vi "TPB Facade.vi"(0 "Data In":T5, 2 "Display State In":T2={"Window Handle"=refnum, "Maximum"=100, "State Change Action"=enum."Method - Initialize", "Running"=FALSE, "Visable Items"={"Label"=TRUE, "Caption"=FALSE}, "Value"=100, "Show Progress Bar"=FALSE}, 3 "Container State":T4) -> (6 "Data Out":T5, 7 "Display State Out":T2={"Window Handle"=refnum, "Maximum"=100, "State Change Action"=enum."Method - Initialize", "Running"=FALSE, "Visable Items"={"Label"=TRUE, "Caption"=FALSE}, "Value"=100, "Show Progress Bar"=FALSE}, 8 "Action":T1)   [LabVIEW 2011, in "Taskbar Progress Bar.xctl"]
uses:
  Taskbar Progress Bar.xctl
  TPB Data.ctl
  <vilib>/_xctls/Container State.ctl
  TPB State.ctl
  TypeDefs/Dispaly State Change Methods.ctl
  <vilib>/_xctls/Action.ctl
  <vilib>/TaskbarProgressAPI/_TypeDefs/Progress State.ctl
  <vilib>/_xctls/XControlSupport.lvlib
  <vilib>/TaskbarProgressAPI/TaskbarProgressAPI.lvlib
panel:
  out "Glyph":u16(ring)
  out "Progress Bar":u64(slide) scale=0.0..100.0
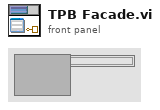
[diagram p1: front panel]
types:
  T1 = typedef "XControlSupport.lvlib/Action.ctl" = cluster{"Data Changed?":bool, "State Changed?":bool, "Action Name":string}
  T2 = typedef "Taskbar Progress Bar.xctl/TPB State.ctl" = cluster{"Window Handle":refnum<k24>, "Maximum":u64, "State Change Action":T3, "Running":bool, "Visable Items":cluster{"Label":bool, "Caption":bool}, "Value":u64, "Show Progress Bar":bool}
  T3 = typedef "Taskbar Progress Bar.xctl/Dispaly State Change Methods.ctl" = enum16{"No Action", "Created", "Method - Initialize", "Method - Increment", "Method - Set Value", "Method - Pause", "Method - Error", "Method - Finish", "Property - Show Progress Bar"}
  T4 = typedef "XControlSupport.lvlib/Container State.ctl" = cluster{"Indicator?":bool, "Run Mode?":bool, " Refnum":refnum<vi>}
  T5 = typedef "Taskbar Progress Bar.xctl/TPB Data.ctl" = u64
  T6 = typedef "TaskbarProgressAPI.lvlib/Progress State.ctl" = i32
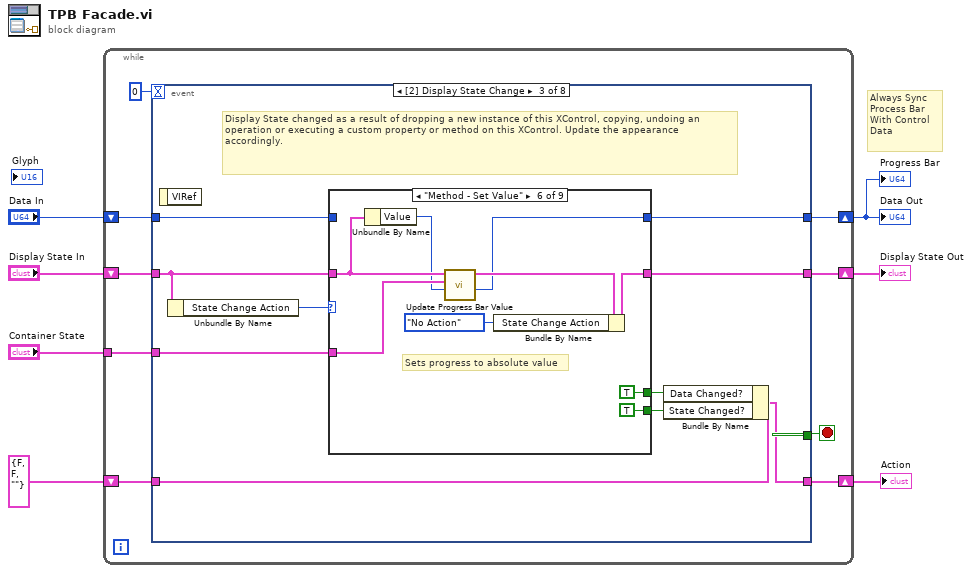
[diagram p0: block diagram]
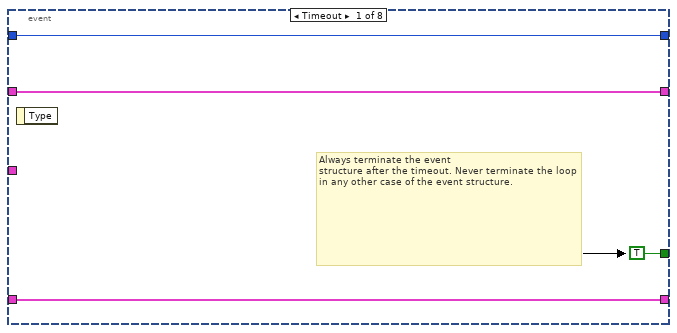
[diagram p2: hidden frame]
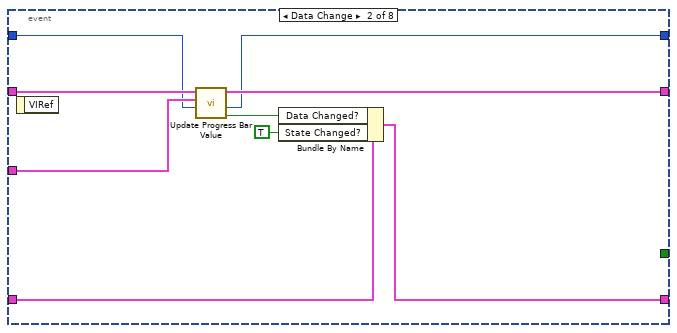
[diagram p3: hidden frame]
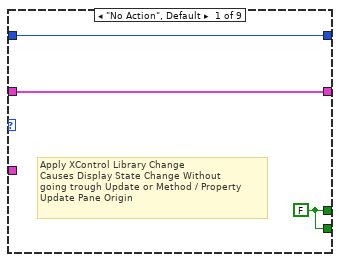
[diagram p4: hidden frame]
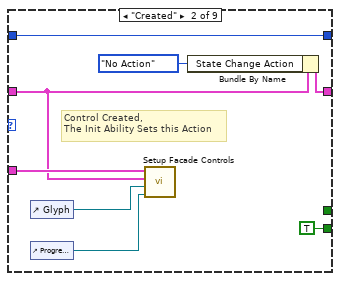
[diagram p5: hidden frame]
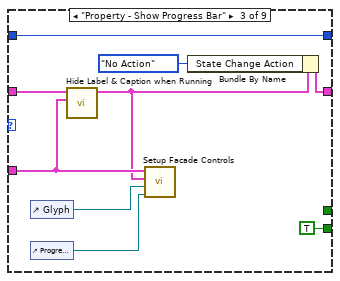
[diagram p6: hidden frame]
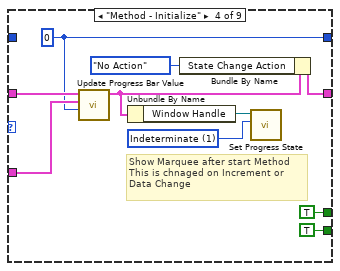
[diagram p7: hidden frame]
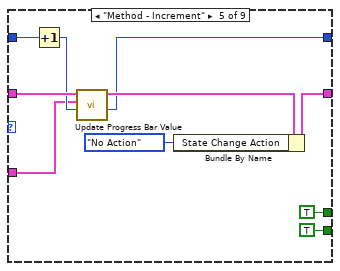
[diagram p8: hidden frame]
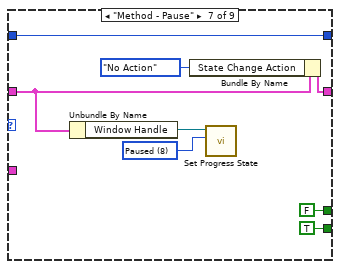
[diagram p9: hidden frame]
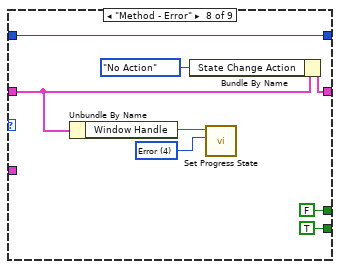
[diagram p10: hidden frame]
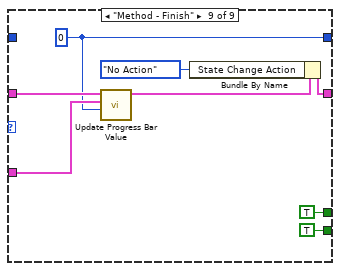
[diagram p11: hidden frame]
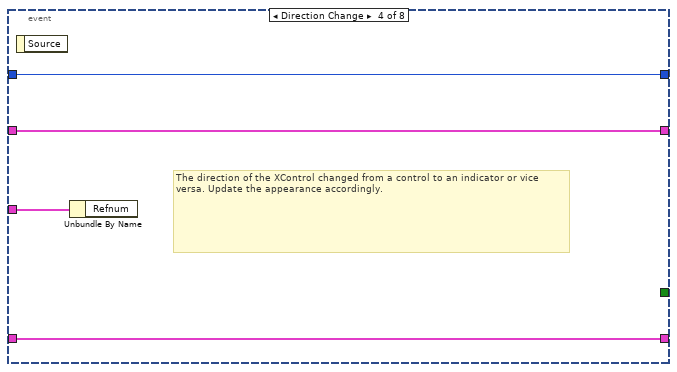
[diagram p12: hidden frame]
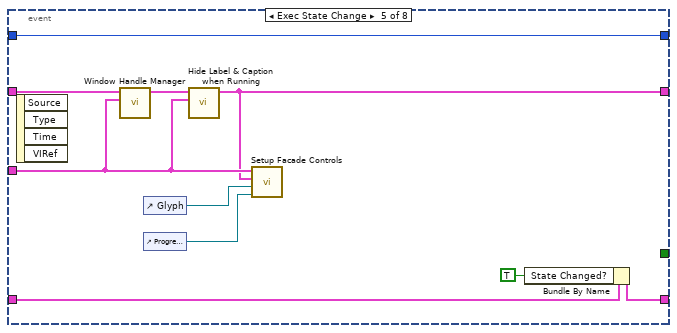
[diagram p13: hidden frame]
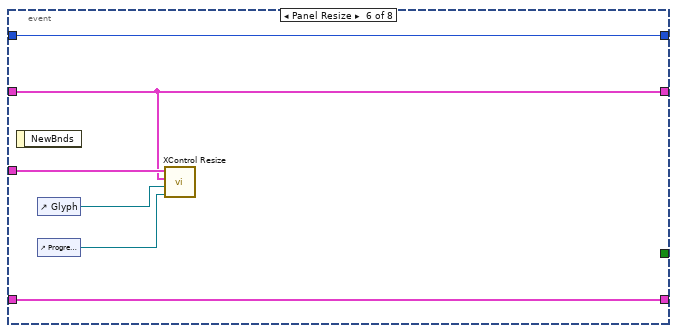
[diagram p14: hidden frame]
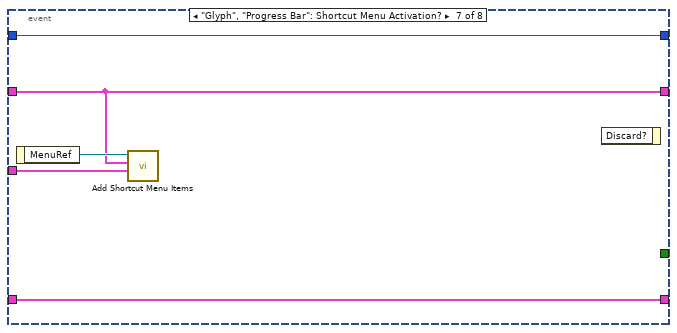
[diagram p15: hidden frame]
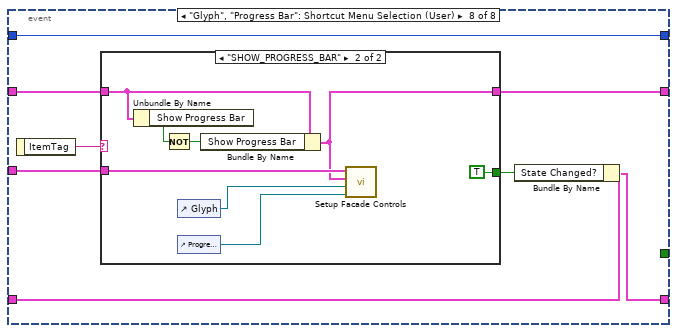
[diagram p16: hidden frame]
diagram:
  # "Always Sync \nProcess Bar\nWith Control \nData"
  n1 = while {
    shift-right: [w15] -> w5
    shift-left: "Display State In" -> [w16]
    tunnel: "Container State" -> [w12]
    shift-right: [w8] -> w1
    shift-left: "Data In" -> [w11]
    shift-right: [w9] -> w3
    shift-left: T1 {"Data Changed?"=FALSE, "State Changed?"=FALSE, "Action Name"=""} ("Action") -> [w10]
    stop <- w14 stop-if-true
    n2 = event shown="[2] Display State Change" {
      selector: _ -> [_ _ _ _ _ _ _ _]
      dyn-events: _ -> [_ _ _ _ _ _ _ _]
      timeout: 0 -> [_ _ _ _ _ _ _ _]
      tunnel: w16 -> [w18 w27 w38 w115 w124 w129 w133 w142]
      tunnel: [w18 w28 w34 w115 w119 w129 w133 w141] -> w15
      tunnel: [TRUE _ _ _ _ _ _ _] -> w14
      tunnel: w12 -> [_ w26 w30 w116 w120 w130 w134 w138]
      tunnel: w11 -> [w17 w25 w36 w114 w126 w131 w137 w145]
      tunnel: [w17 w21 w35 w114 w126 w131 w137 w145] -> w8
      tunnel: [w19 w24 w33 w113 w123 w132 w136 w140] -> w9
      tunnel: w10 -> [w19 w29 w39 w113 w125 w132 w136 w144]
      event Timeout {
        # "Always terminate the event\nstructure after the timeout. Never terminate the loop in any other case of the event structure."
        n3 = event-data() -> ()  [unwired: 1 in, 1 out]
      }
      event Data Change {
        n4 = event-data() -> ()  [unwired: 1 in, 1 out]
        n5 = call "Update Progress Bar Value.vi"("Data in"=w25, "Container State"=w26, "Display State in"=w27) -> ("Coerced?"=w22:bool, "Data Out"=w21:T5, "Display State out"=w28:T2)  [unwired: 6 in]
        n6 = Bundle By Name(cluster=w29, "Data Changed?"=w22, "State Changed?"=TRUE) -> (w24:T1)
      }
      event Display State Change {
        # "Display State changed as a result of dropping a new instance of this XControl, copying, undoing an operation or executing a custom property or method on this XControl. Update the appearance accordingly."
        n7 = event-data() -> ()  [unwired: 1 in, 1 out]
        n8 = Unbundle By Name(w38) -> ("State Change Action"=w37:T3)
        n9 = case shown="\"Method - Set Value\"" w37 {
          tunnel: w38 -> [w41 w45 w53 w65 w74 w81 w91 w99 w108]
          tunnel: w36 -> [w42 w49 w58 _ w79 _ w92 w100 _]
          tunnel: [w42 w49 w58 w63 w70 w82 w92 w100 w105] -> w35
          tunnel: [w41 w48 w57 w68 w76 w86 w94 w102 w110] -> w34
          tunnel: [w40 TRUE TRUE TRUE TRUE TRUE TRUE TRUE TRUE] -> w32
          tunnel: [w40 _ _ TRUE TRUE TRUE FALSE FALSE TRUE] -> w31
          tunnel: w30 -> [_ w46 w52 w64 w72 w84 _ _ w107]
          frame "No Action", Default {
            w40 = FALSE
            # "Apply XControl Library Change\nCauses Display State Change Without \ngoing trough Update or Method / Property\nUpdate Pane Origin"
          }
          frame "Created" {
            # "Control Created,\nThe Init Ability Sets this Action"
            n10 = control-ref of="Glyph"() -> (w44:refnum<vi>)
            n11 = control-ref of="Progress Bar"() -> (w43:refnum<vi>)
            n12 = call "Setup Facade Controls.vi"("Progress Bar Refnum"=w43, "Glyph Refnum"=w44, "State"=w45, "Container State"=w46) -> ()  [unwired: 8 in]
            n13 = Bundle By Name(cluster=w45, "State Change Action"=Dispaly_State_Change_Methods."No Action") -> (w48:T2)
          }
          frame "Property - Show Progress Bar" {
            n14 = control-ref of="Glyph"() -> (w55:refnum<vi>)
            n15 = control-ref of="Progress Bar"() -> (w54:refnum<vi>)
            n16 = call "Hide Label & Caption when Running.vi"("Container State"=w52, "Display State out in"=w53) -> ("Display State out out"=w51:T2)  [unwired: 9 in]
            n17 = call "Setup Facade Controls.vi"("Progress Bar Refnum"=w54, "Glyph Refnum"=w55, "State"=w51, "Container State"=w52) -> ()  [unwired: 8 in]
            n18 = Bundle By Name(cluster=w51, "State Change Action"=Dispaly_State_Change_Methods."No Action") -> (w57:T2)
          }
          frame "Method - Initialize" {
            w60 = T6 1 items=["NoProgress"=0, "Indeterminate"=1, "Normal"=2, "Error"=4, "Paused"=8] ("State (No Progress)")
            w63 = T5 0 ("Data in")
            # "Show Marquee after start Method\nThis is chnaged on Increment or\nData Change"
            n19 = call "Update Progress Bar Value.vi"("Data in"=w63, "Container State"=w64, "Display State in"=w65) -> ("Display State out"=w62:T2)  [unwired: 6 in, 2 out]
            n20 = Unbundle By Name(w62) -> ("Window Handle"=w61:refnum<k24>)
            n21 = Bundle By Name(cluster=w62, "State Change Action"=Dispaly_State_Change_Methods."No Action") -> (w68:T2)
            n22 = call <vilib>:"Set Progress State.vi"("State (No Progress)"=w60, "Window Handle"=w61) -> ()  [unwired: 8 in, 2 out]
          }
          frame "Method - Increment" {
            n23 = Increment(x=w79) -> (x+1=w73:T5)
            n24 = call "Update Progress Bar Value.vi"("Data in"=w73, "Container State"=w72, "Display State in"=w74) -> ("Data Out"=w70:T5, "Display State out"=w71:T2)  [unwired: 6 in, 1 out]
            n25 = Bundle By Name(cluster=w71, "State Change Action"=Dispaly_State_Change_Methods."No Action") -> (w76:T2)
          }
          frame "Method - Set Value" {
            # "Sets progress to absolute value"
            n26 = Unbundle By Name(w81) -> ("Value"=w80:u64)
            n27 = call "Update Progress Bar Value.vi"("Data in"=w80, "Container State"=w84, "Display State in"=w81) -> ("Data Out"=w82:T5, "Display State out"=w83:T2)  [unwired: 6 in, 1 out]
            n28 = Bundle By Name(cluster=w83, "State Change Action"=Dispaly_State_Change_Methods."No Action") -> (w86:T2)
          }
          frame "Method - Pause" {
            w89 = T6 8 items=["NoProgress"=0, "Indeterminate"=1, "Normal"=2, "Error"=4, "Paused"=8] ("State (No Progress)")
            n29 = Unbundle By Name(w91) -> ("Window Handle"=w90:refnum<k24>)
            n30 = Bundle By Name(cluster=w91, "State Change Action"=Dispaly_State_Change_Methods."No Action") -> (w94:T2)
            n31 = call <vilib>:"Set Progress State.vi"("State (No Progress)"=w89, "Window Handle"=w90) -> ()  [unwired: 8 in, 2 out]
          }
          frame "Method - Error" {
            w97 = T6 4 items=["NoProgress"=0, "Indeterminate"=1, "Normal"=2, "Error"=4, "Paused"=8] ("State (No Progress)")
            n32 = Unbundle By Name(w99) -> ("Window Handle"=w98:refnum<k24>)
            n33 = Bundle By Name(cluster=w99, "State Change Action"=Dispaly_State_Change_Methods."No Action") -> (w102:T2)
            n34 = call <vilib>:"Set Progress State.vi"("State (No Progress)"=w97, "Window Handle"=w98) -> ()  [unwired: 8 in, 2 out]
          }
          frame "Method - Finish" {
            w105 = T5 0
            n35 = call "Update Progress Bar Value.vi"("Data in"=w105, "Container State"=w107, "Display State in"=w108) -> ("Display State out"=w106:T2)  [unwired: 6 in, 2 out]
            n36 = Bundle By Name(cluster=w106, "State Change Action"=Dispaly_State_Change_Methods."No Action") -> (w110:T2)
          }
        }
        n37 = Bundle By Name(cluster=w39, "Data Changed?"=w31, "State Changed?"=w32) -> (w33:T1)
      }
      event Direction Change {
        # "The direction of the XControl changed from a control to an indicator or vice versa. Update the appearance accordingly."
        n38 = event-data() -> ()  [unwired: 1 in, 1 out]
        n39 = Unbundle By Name(w116) -> ()  [unwired: 1 out]
      }
      event Exec State Change {
        n40 = event-data() -> ()  [unwired: 1 in, 4 out]
        n41 = call "Window Handle Manager.vi"("Container State"=w120, "Display State in"=w124) -> ("Display State out"=w121:T2)  [unwired: 9 in]
        n42 = control-ref of="Glyph"() -> (w118:refnum<vi>)
        n43 = control-ref of="Progress Bar"() -> (w117:refnum<vi>)
        n44 = call "Hide Label & Caption when Running.vi"("Container State"=w120, "Display State out in"=w121) -> ("Display State out out"=w119:T2)  [unwired: 9 in]
        n45 = call "Setup Facade Controls.vi"("Progress Bar Refnum"=w117, "Glyph Refnum"=w118, "State"=w119, "Container State"=w120) -> ()  [unwired: 8 in]
        n46 = Bundle By Name(cluster=w125, "State Changed?"=TRUE) -> (w123:T1)
      }
      event Panel Resize {
        n47 = event-data() -> ()  [unwired: 1 in, 1 out]
        n48 = control-ref of="Glyph"() -> (w128:refnum<vi>)
        n49 = control-ref of="Progress Bar"() -> (w127:refnum<vi>)
        n50 = call "XControl Resize.vi"("Progress Bar Refnum"=w127, "Glyph Refnum"=w128, "State"=w129, "Container State"=w130) -> ()  [unwired: 8 in]
      }
      event "Glyph", "Progress Bar": Shortcut Menu Activation? {
        n51 = event-data() -> ("MenuRef"=w135:refnum<k9>)  [unwired: 1 in]
        n52 = call "Add Shortcut Menu Items.vi"("Container State"=w134, "Display State In"=w133, "Menu in"=w135) -> ()  [unwired: 9 in]
        n53 = event-data() -> ()  [unwired: 2 in, 1 out]
      }
      event "Glyph", "Progress Bar": Shortcut Menu Selection (User) {
        n54 = event-data() -> ("ItemTag"=w143:string)  [unwired: 1 in]
        n55 = case shown="\"SHOW_PROGRESS_BAR\"" w143 {
          tunnel: w142 -> [w146 w153]
          tunnel: [w146 w149] -> w141
          tunnel: [_ TRUE] -> w139
          tunnel: w138 -> [_ w150]
          frame Default {
          }
          frame "SHOW_PROGRESS_BAR" {
            n56 = Unbundle By Name(w153) -> ("Show Progress Bar"=w154:bool)
            n57 = Not(x=w154) -> (.not. x?=w152:bool)
            n58 = control-ref of="Glyph"() -> (w148:refnum<vi>)
            n59 = control-ref of="Progress Bar"() -> (w147:refnum<vi>)
            n60 = Bundle By Name(cluster=w153, "Show Progress Bar"=w152) -> (w149:T2)
            n61 = call "Setup Facade Controls.vi"("Progress Bar Refnum"=w147, "Glyph Refnum"=w148, "State"=w149, "Container State"=w150) -> ()  [unwired: 8 in]
          }
        }
        n62 = Bundle By Name(cluster=w144, "State Changed?"=w139) -> (w140:T1)
      }
    }
  }
  "Display State Out" <- w5
  "Data Out" <- w1
  "Action" <- w3
  "Progress Bar" <- w1
